vi "Rotation3d_Plus.vi"(9 "other Rotation3d":T1={"Q_quaternion"={"R"=1.0, "V"=[0.0, 0.0, 0.0]}}, 11 "in Rotation3d":T1={"Q_quaternion"={"R"=1.0, "V"=[0.0, 0.0, 0.0]}}) -> (3 "out Rotation3d":T1={"Q_quaternion"={"R"=1.0, "V"=[0.0, 0.0, 0.0]}})   [LabVIEW 2019, in "Trajectory_Library.lvlib"]
doc: "Adds two rotations together.\n\nThis function is the same as RotateBy.\n\nParameters:\n\n - IN ROTATION3D - This rotation data structure\n - OTHER ROTATION3D - The rotation to add.\n\nReturns:\n- OUT ROTATION3D - The sum of the two rotations."
uses:
  Trajectory_Library.lvlib
  TypeDef/QUATERNION.ctl
  TypeDef/ROTATION3D.ctl
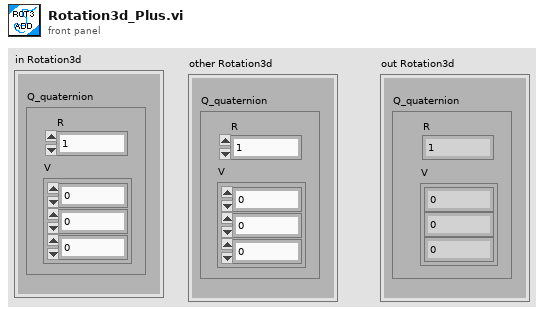
[diagram p1: front panel]
types:
  T1 = typedef "Trajectory_Library.lvlib/ROTATION3D.ctl" = cluster{"Q_quaternion":T2}
  T2 = typedef "Trajectory_Library.lvlib/QUATERNION.ctl" = cluster{"R":dbl, "V":dbl[]}
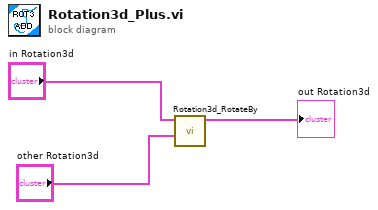
[diagram p0: block diagram]
diagram:
  n1 = call "Rotation3d_RotateBy.vi"("other Rotation3d"="other Rotation3d", "in Rotation3d"="in Rotation3d") -> ("out Rotation3d"=→"out Rotation3d":T1)  [unwired: 9 in]
